vi "UT - File Exists.vi"() -> (0 "error out":errorcluster)   [LabVIEW 2019, in "HDF5 Tools.lvlib"]
uses:
  HDF5 Tools.lvlib
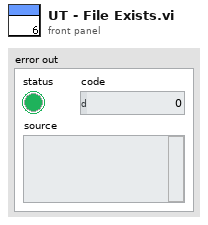
[diagram p1: front panel]
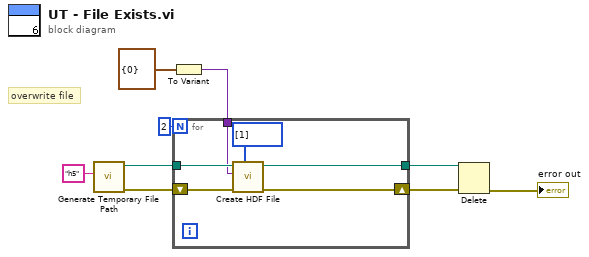
[diagram p0: block diagram]
diagram:
  # "overwrite file"
  n1 = call <vilib>:"Generate Temporary File Path.vi"("Temporary File Extension (tmp)"="h5") -> ("error out"=w8:errorcluster, "Unique Temporary File Path"=w7:path)  [unwired: 9 in]
  n2 = To Variant(anything=cluster{"Value":i32} {"Value"=0}) -> (Variant=w1:variant)
  n3 = for {
    N: 2 -> [_]
    shift-right: [w13] -> w6
    shift-left: w8 -> [w15]
    tunnel: w7 -> [w14]
    tunnel: [w12] -> w5
    tunnel: w1 -> [w11]
    n4 = call "Create HDF File.vi"("Dims"=u64[] [1], "error in (no error)"=w15, "variant"=w11, "path"=w14) -> ("error out"=w13:errorcluster, "path out"=w12:path)  [unwired: 5 in, 1 out]
  }
  n5 = Delete(path (use dialog)=w5, error in=w6) -> (error out=→"error out":errorcluster)  [unwired: 3 in, 2 out]
